vi "Cluster2Str.vi"(3 "error in (no error)":errorcluster, 5 "Data_Cluster":variant) -> (0 "error out":errorcluster, 2 "Formatted data out":string)   [LabVIEW 2019, in "Tools.lvlib"]
doc: "Use this VI to change any data into a string."
uses:
  Tools.lvlib
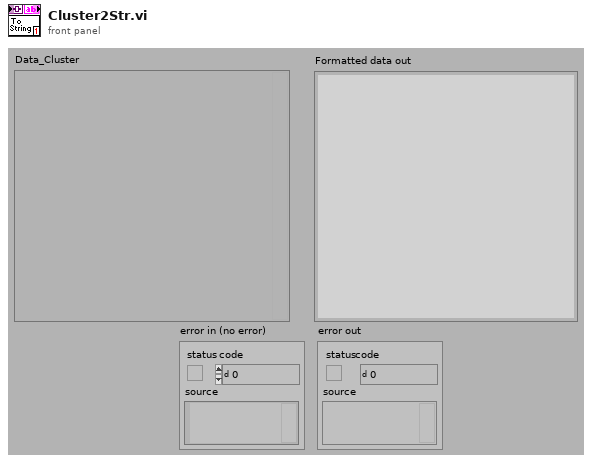
[diagram p1: front panel]
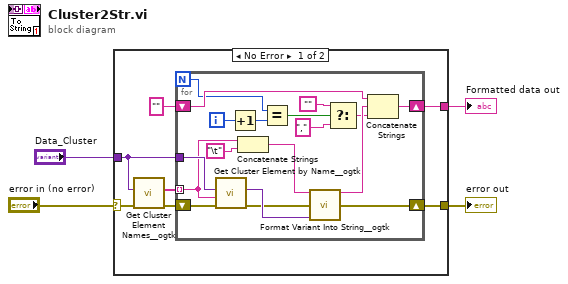
[diagram p0: block diagram]
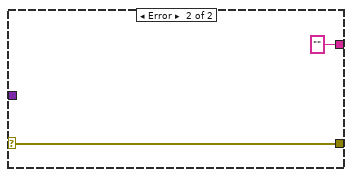
[diagram p2: hidden frame]
diagram:
  n1 = case shown="No Error" "error in (no error)" {
    selector: "error in (no error)" -> [w5 w31]
    tunnel: [w9 w31] -> w3
    tunnel: [w8 ""] -> w1
    tunnel: "Data_Cluster" -> [w7 _]
    frame No Error {
      n2 = call <userlib>:"Get Cluster Element Names__ogtk.vi"("error in (no error)"=w5, "Cluster"=w7) -> ("error out"=w6:errorcluster, "Element Names"=w10:string[])  [unwired: 8 in]
      n3 = for {
        N -> [w18]
        tunnel: w10 -> [w26] mode=indexing
        tunnel: w7 -> [w29]
        shift-right: [w25] -> w9
        shift-left: w6 -> [w20]
        shift-right: [w22] -> w8
        shift-left: "" -> [w21]
        i -> [w17]
        n4 = call <userlib>:"Get Cluster Element by Name__ogtk.vi"("error in (no error)"=w20, "Element Name"=w26, "Cluster"=w29) -> ("error out"=w19:errorcluster, "VElement"=w28:variant)  [unwired: 6 in, 1 out]
        n5 = Increment(x=w17) -> (x+1=w16:i32)
        n6 = Concatenate Strings(w26, "\t") -> (w24:string)
        n7 = Equal?(x=w18, y=w16) -> (x = y?=w15:bool)
        n8 = call <userlib>:"Format Variant Into String__ogtk.vi"("Input String"=w24, "error in (no error)"=w19, "Variant"=w28) -> ("Output String"=w23:string, "error out"=w25:errorcluster)  [unwired: 11 in]
        n9 = Select(t="", s=w15, f="," ("string")) -> (s? t:f=w13:string)
        n10 = Concatenate Strings(w21, w23, w13) -> (w22:string)
      }
    }
    frame Error {
    }
  }
  "error out" <- w3
  "Formatted data out" <- w1
